vi "Act on Action_Do.vi"(8 "error in (no error)":errorcluster, 10 "Project Builder in":refnum<class "Project Builder.lvclass">, 11 "Project Action in":refnum<class "Project Action.lvclass">) -> (0 "error out":errorcluster, 1 "Success?":bool, 2 "Project Builder out":refnum<class "Project Builder.lvclass">, 3 "Report":refnum<class "Report Data.lvclass">)   [LabVIEW 2019, in "ProjectBuilder.lvlib" / "Project Builder.lvclass"]
doc: "Specify how the Project Builder should act on Project Actions.\n\nThe default implementation functions as a wrapper for 'Run Action_Do.vi'."
uses:
  Project Builder.lvclass
  Project Action/Project Action.lvclass
  Data/Report Data/Report Data.lvclass
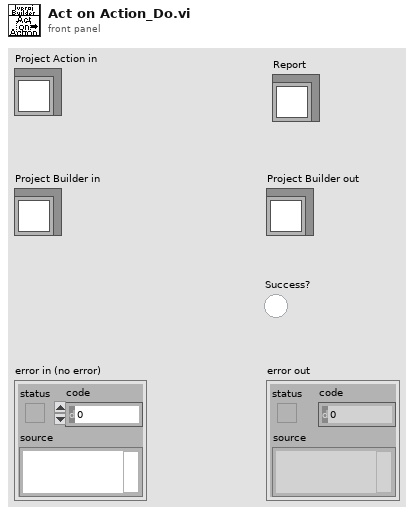
[diagram p1: front panel]
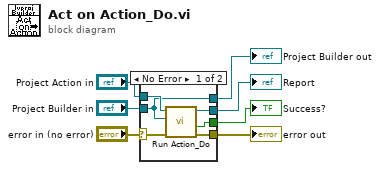
[diagram p0: block diagram]
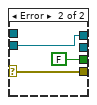
[diagram p2: hidden frame]
diagram:
  n1 = case shown="No Error" "error in (no error)" {
    selector: "error in (no error)" -> [w10 w16]
    tunnel: [w9 w16] -> w6
    tunnel: [w11 w15] -> w4
    tunnel: "Project Builder in" -> [w11 w15]
    tunnel: [w12 FALSE] -> w3
    tunnel: "Project Action in" -> [w13 _]
    tunnel: [w8 _] -> w1
    frame No Error {
      n2 = call-dynamic "Run Action_Do.vi"("error in (no error)"=w10, "Project Builder in"=w11, "Project Action"=w13) -> ("error out"=w9:errorcluster, "Success?"=w12:bool, "Report"=w8:refnum<class "Report Data.lvclass">)  [unwired: 6 in]
    }
    frame Error {
    }
  }
  "error out" <- w6
  "Project Builder out" <- w4
  "Success?" <- w3
  "Report" <- w1
